vi "buffor_x.vi"() -> ()   [LabVIEW 2021]
panel:
  out "Waveform Chart":cluster{"element":dbl, "Xwe":dbl}(graph)
  out "Xwy":dbl
  in  "stop":bool
  out "Bufor":dbl[](array[numeric])
  out "equal to delay?":bool
  out "default result":i32
  out "larger than delay?":bool
  in  "delay":i32
  in  "Xwe":dbl
  in  "element":dbl
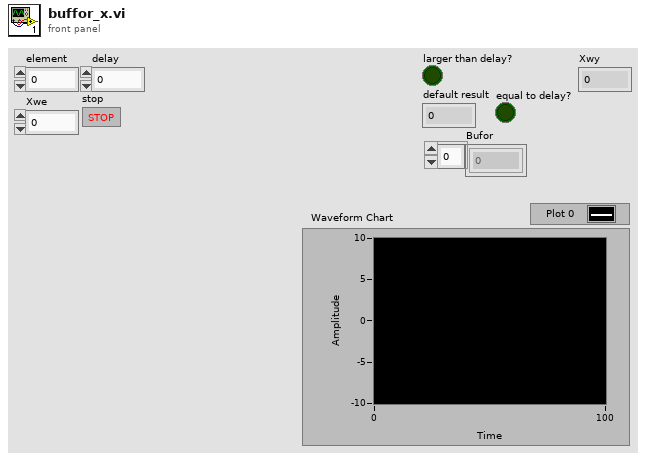
[diagram p1: front panel]
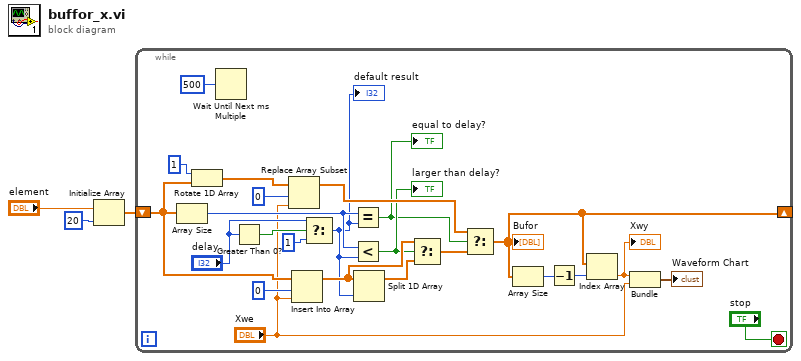
[diagram p0: block diagram]
diagram:
  n1 = Initialize Array("element", 20 ("dimension size")) -> (w1:dbl[])
  n2 = while {
    shift-right: [w9] -> _
    shift-left: w1 -> [w18]
    stop <- "stop" stop-if-true
    n3 = Array Size(array=w18) -> (size(s)=w13:i32)
    n4 = Rotate 1D Array(1:w18, 2:1 ("n")) -> (0:w25:dbl[])
    n5 = Wait Until Next ms Multiple(millisecond multiple=u32 500) -> ()  [unwired: 1 out]
    n6 = Greater Than 0?(x="delay") -> (x > 0?=w17:bool)
    n7 = Replace Array Subset(array=w25, new element="Xwe", index=0) -> (w20:dbl[])
    n8 = Insert Into Array(array=w18, index=0, new element="Xwe") -> (w21:dbl[])
    n9 = Select(t="delay", s=w17, f=1) -> (s? t:f=w12:i32)
    "default result" <- w12
    n10 = Equal?(x=w13, y=w12) -> (x = y?=w11:bool)
    "equal to delay?" <- w11
    n11 = Less?(x=w13, y=w12) -> (x < y?=w14:bool)
    "larger than delay?" <- w14
    n12 = Split 1D Array(array=w21, index=w12) -> (first subarray=w22:dbl[])  [unwired: 1 out]
    n13 = Select(t=w21, s=w14, f=w22) -> (s? t:f=w19:dbl[])
    n14 = Select(t=w20, s=w11, f=w19) -> (s? t:f=w9:dbl[])
    "Bufor" <- w9
    n15 = Array Size(array=w9) -> (size(s)=w8:i32)
    n16 = Decrement(x=w8) -> (x-1=w7:i32)
    n17 = Index Array(array=w9, index=w7) -> (element=w6:dbl)
    "Xwy" <- w6
    n18 = Bundle("element"=w6, "Xwe"="Xwe") -> (→"Waveform Chart":cluster{"element":dbl, "Xwe":dbl})  [unwired: 1 in]
  }
